vi "main_ctrl.vi"(8 "error in":errorcluster) -> (0 "error out":errorcluster caption="Error")   [LabVIEW 2014]
uses:
  <vilib>/Rock Robotics/WPI/DriverStation/WPI_DriverStationRobotMode2.ctl
  typedefs/test/test data.ctl
  typedefs/test/test controls.ctl
  typedefs/fg_getset.ctl
  typedefs/vision/vision enable.ctl
  typedefs/state machine/subStates.ctl
  typedefs/state machine/singleUseSubstate.ctl
  <vilib>/Rock Robotics/WPI/RobotDrive/WPI_RobotDriveGetSetRefNum.vi
  typedefs/vision/vision data.ctl
  global variables/vision.vi
panel:
  out "vision errors":errorcluster
  in  "Test\nControls":T1 {"Slider" scale=-1.0..1.0}
  out "Test Data":T2
  out "Robot Mode":T3
  out "Vision mSPI":u32
  out "Vision IPS":dbl
  out "Main IPS":dbl
  out "Main mSPI":u32
  # "Test Input/Output"
  # "MAIN CONTROL"
  # "holds robot control code - dual parallel state machine"
  # "mSPI: milliseconds per iteration\nIPS: iterations per second"
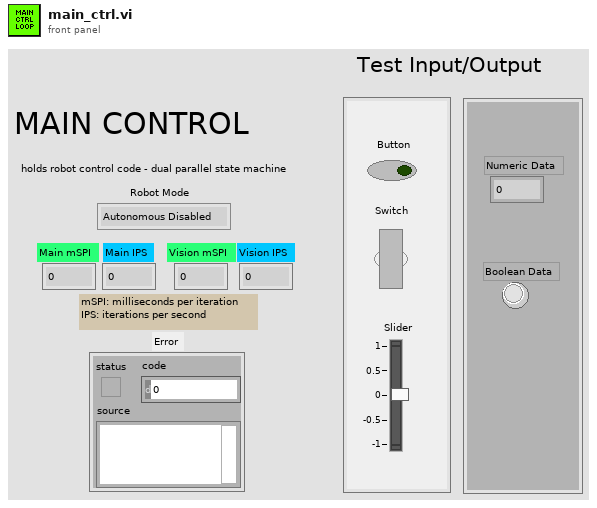
[diagram p1: front panel]
types:
  T1 = typedef "test controls.ctl" = cluster{"Button":bool, "Switch":bool, "Slider":dbl}
  T2 = typedef "test data.ctl" = cluster{"Numeric Data":dbl, "Boolean Data":bool}
  T3 = typedef "WPI_DriverStationRobotMode2.ctl" = enum16{"Autonomous Disabled", "Autonomous Enabled", "Teleop Disabled", "Teleop Enabled", "Disconnected", "Finish", "Test Disabled", "Test Enabled", "Emergency Stopped"}
  T4 = typedef "fg_getset.ctl" = enum16{"Get", "Set"}
  T5 = typedef "vision data.ctl" = cluster{"x":dbl, "y":dbl, "area":dbl, "width":dbl, "height":dbl}
  T6 = typedef "vision enable.ctl" = enum16{"Enable", "Disable", "Stop"}
  T7 = typedef "WPI_CameraDevRef.ctl" = cluster{"Camera Address":string, "CameraStatus":errorcluster}
  T8 = typedef "IMAQ Image.ctl" = refnum<image>
  T9 = typedef "WPI_RobotDriveDevRef.ctl" = cluster{"DevStatus":errorcluster, "Motors[]":T10[], "Square Inputs":bool, "Max Output":dbl}
  T10 = typedef "WPI_MotorControlDeviceRef.ctl" = cluster{"DeviceStatus":errorcluster, "Type":T11, "PWM":cluster{"Controller":T12, "PWM Channel":T13, "DeadBand":T14}, "CAN":cluster{"Device Number":u8, "Control Mode":T15, "Semaphore":T16, "Max Vout":dbl, "TalonSRX Control Mode":T17}, "Invert":bool, "TransformRef":T18, "InvTransformRef":T18}
  T11 = typedef "WPI_MotorControlType.ctl" = enum16{"PWM", "CAN", "CANTalonSRX"}
  T12 = typedef "FPGA_TypedefDigitalModule.ctl" = enum16{"Controller 1"}
  T13 = typedef "FPGA_DIOPWMChannel.ctl" = enum8{"PWM 0", "PWM 1", "PWM 2", "PWM 3", "PWM 4", "PWM 5", "PWM 6", "PWM 7", "PWM 8", "PWM 9", "PWM MXP 0", "PWM MXP 1", "PWM MXP 2", "PWM MXP 3", "PWM MXP 4", "PWM MXP 5", "PWM MXP 6", "PWM MXP 7", "PWM MXP 8", "PWM MXP 9", "Invalid"}
  T14 = typedef "WPI_PWMDeadband.ctl" = cluster{"Name":string, "maxPositivePwm":i32, "minPositivePwm":i32, "centerPwm":i32, "maxNegativePwm":i32, "minNegativePwm":i32, "angularRange":u16}
  T15 = typedef "WPI_CANJaguar_ControlMode.ctl" = enum8{"Percent VBus", "Current", "Speed", "Position", "Voltage"}
  T16 = typedef "Semaphore RefNum" = refnum<k1>
  T17 = typedef "WPI_CANTalonSRX_APIControlMode.ctl" = enum8{"Percent VBus", "Speed", "Position", "Slave", "Unchanged / Invalid"}
  T18 = typedef "WPI_PWMTransform_ConPane.ctl" = refnum<vi>
  T19 = typedef "singleUseSubstate.ctl" = enum16{"null", "wait", "open", "close", "end"}
  T20 = typedef "WPI_DriverStationDerivedRobotMode.ctl" = enum16{"Init", "Execute", "Stop"}
  T21 = typedef "subStates.ctl" = enum16{"null", "wait", "driver control", "auto", "manual override", "hold position", "rotate", "intake", "deposit", "test", "end"}
  T22 = typedef "Loop 2 Datatype.ctl" = cluster{"State":T21, "Waiting Loop":i32, "State to Wait For":i32, "Loop ID":i32, "Exit Value":i32}
  T23 = typedef "Loop 1 Datatype.ctl" = cluster{"State":T21, "Waiting Loop":i32, "State to Wait For":i32, "Loop ID":i32, "Exit Value":i32, "Joystick Y":dbl}
  T24 = typedef "Loop 3 Datatype.ctl" = cluster{"State":T21, "Waiting Loop":i32, "State to Wait For":i32, "Loop ID":i32, "Exit Value":i32, "Speed":dbl}
  T25 = typedef "Loop 0 Datatype.ctl" = cluster{"State":T21, "Waiting Loop":i32, "State to Wait For":i32, "Loop ID":i32, "Exit Value":i32, "X Axis":dbl, "Y Axis":dbl, "Center":dbl, "Mode":enum16{"Arcade Drive", "H-Drive"}}
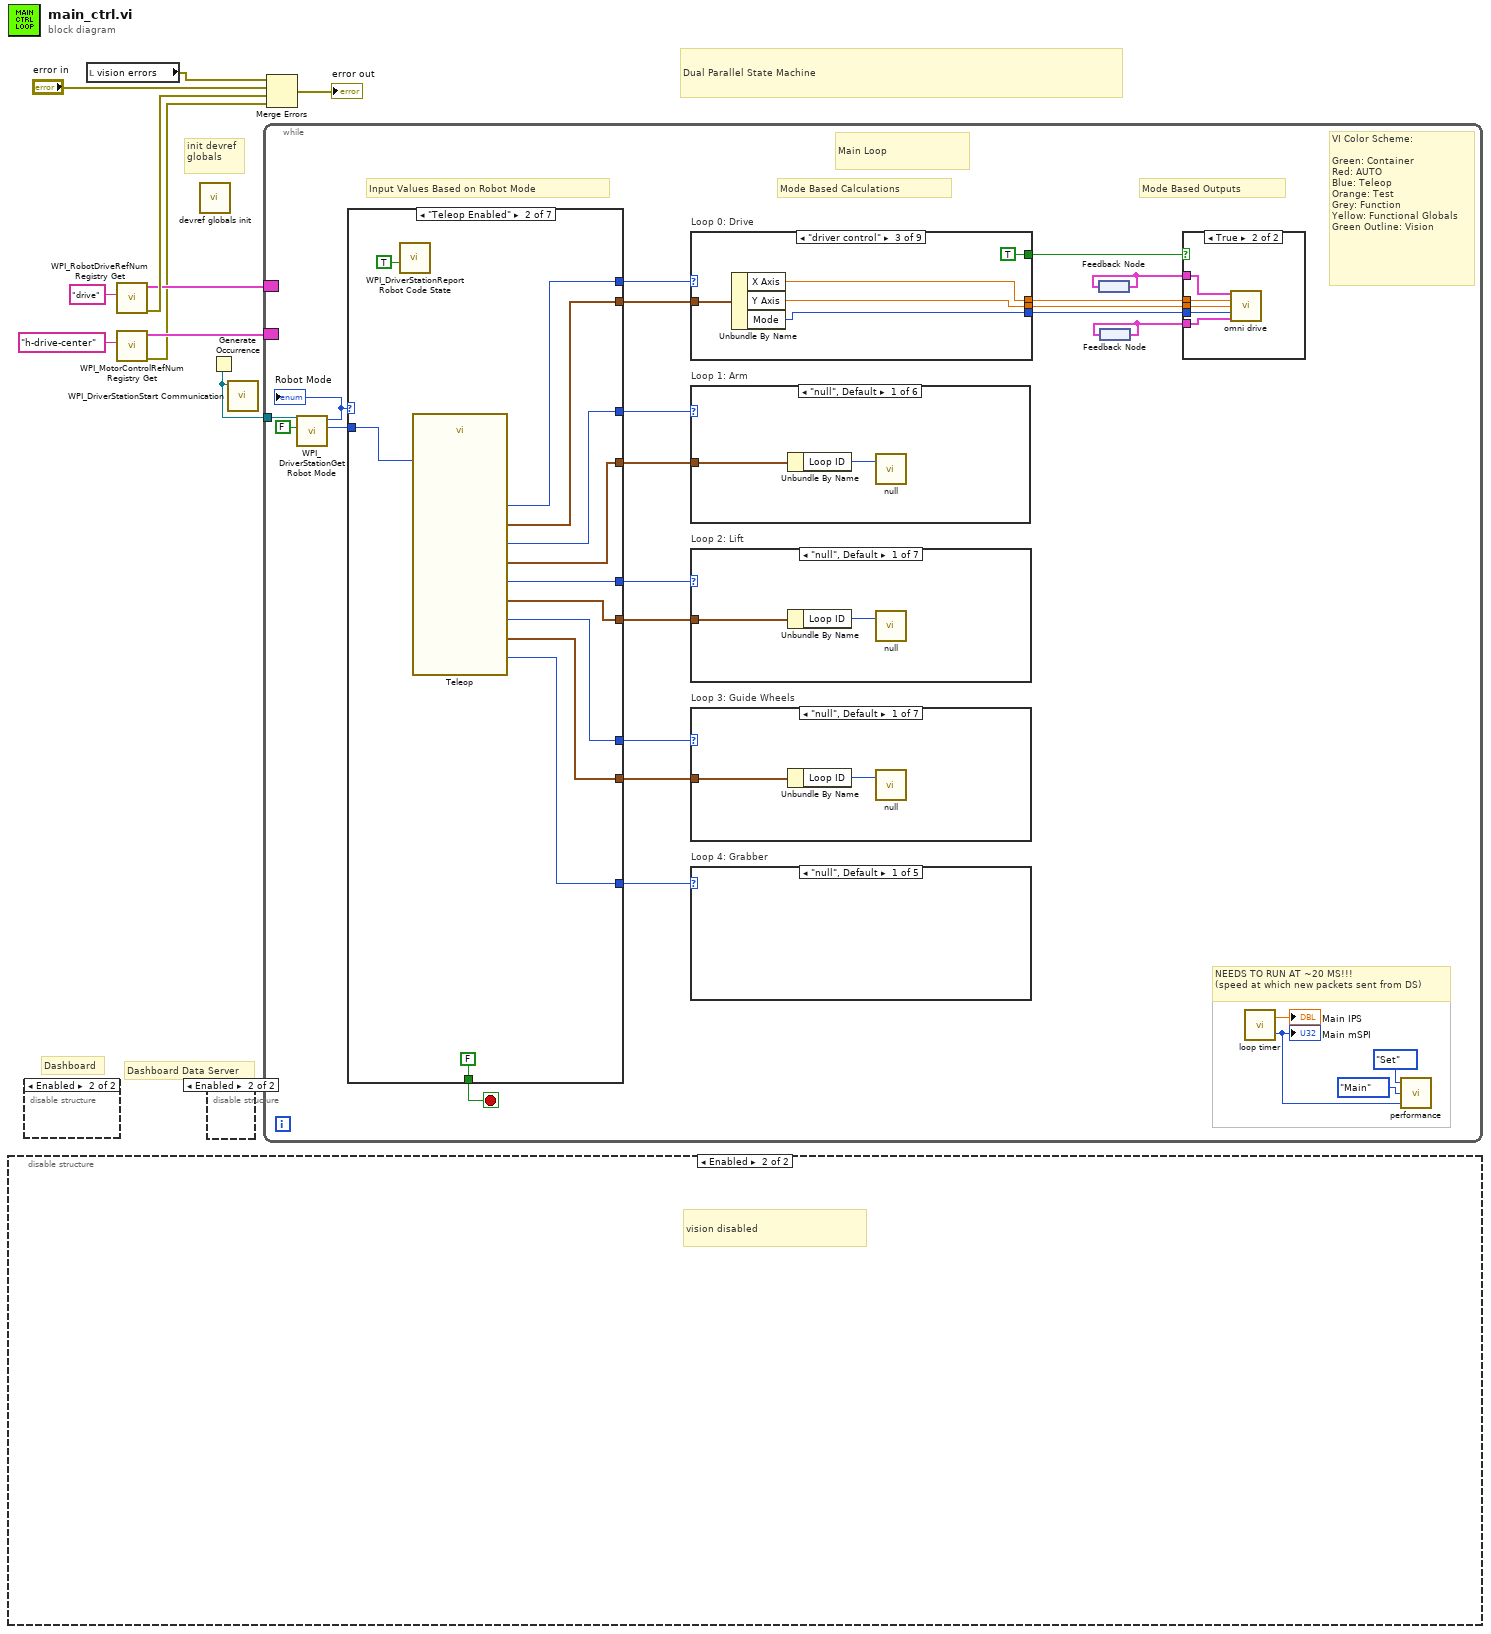
[diagram p0: block diagram]
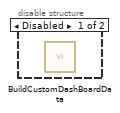
[diagram p2: hidden frame]
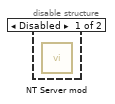
[diagram p3: hidden frame]
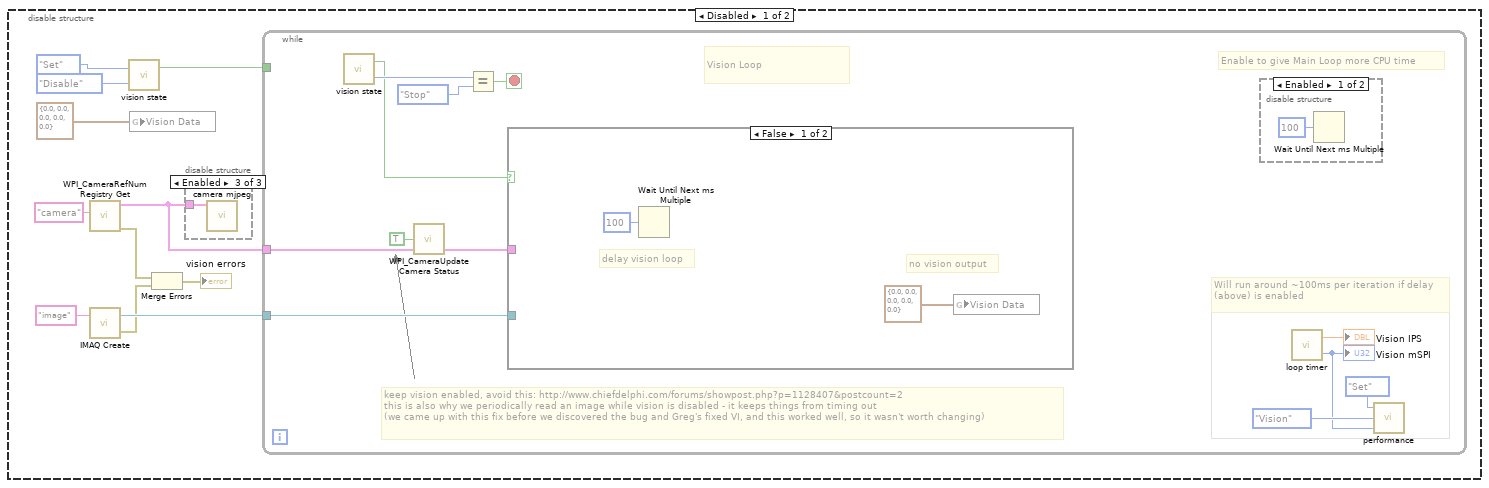
[diagram p4: hidden frame]
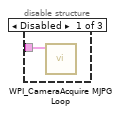
[diagram p5: hidden frame]
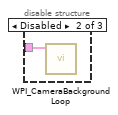
[diagram p6: hidden frame]
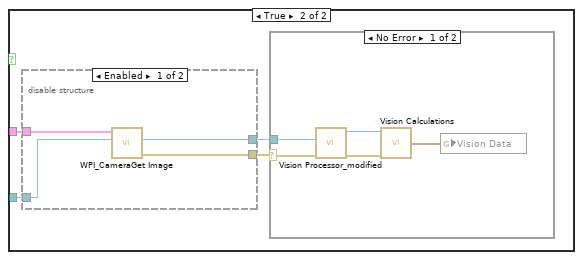
[diagram p8: hidden frame]
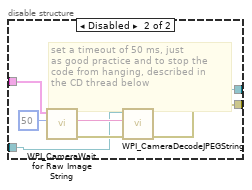
[diagram p10: hidden frame]
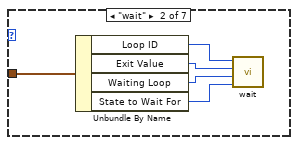
[diagram p15: hidden frame]
diagram:
  # "Dashboard"
  # "init devref\nglobals"
  # "Dual Parallel State Machine"
  # "Dashboard Data Server"
  n1 = disable-structure shown="Enabled" {
    frame Disabled {
      n2 = call <vilib>:"WPI_CameraRefNum Registry Get.vi"("refnum name"="camera") -> ("error out"=w15:errorcluster, "CameraDevRef"=w18:T7)  [unwired: 9 in]
      n3 = call "IMAQ Create"("Image Name"="image") -> ("New Image"=w21:T8, "error out"=w16:errorcluster)  [unwired: 4 in]
      n4 = call "vision state.vi"("State In"=vision_enable."Disable" ("Action"), "Menu"=fg_getset."Set") -> ("Enabled?"=w20:bool)  [unwired: 1 out]
      n5 = global write "vision.vi" "Vision Data"(T5 {"x"=0.0, "y"=0.0, "area"=0.0, "width"=0.0, "height"=0.0} ("Cluster")) -> ()
      n6 = Merge Errors(w15, w16) -> (→"vision errors":errorcluster)
      n7 = disable-structure shown="Enabled" {
        disable-tunnel: w18 -> [w22 w23 w24]
        frame Disabled {
          n8 = call <vilib>:"WPI_CameraAcquire MJPG Loop.vi"("CameraDevRef"=w22) -> ()  [unwired: 11 in]
        }
        frame Disabled {
          n9 = call <vilib>:"WPI_CameraBackground Loop.vi"("CameraDevRef"=w23) -> ()  [unwired: 11 in]
        }
        frame Enabled {
          n10 = call "camera mjpeg.vi"("CameraDevRef"=w24) -> ()  [unwired: 11 in]
        }
      }
      n11 = while {
        tunnel: w21 -> [w35]
        tunnel: w18 -> [w34]
        tunnel: w20 -> [_]
        stop <- w36 stop-if-true
        # "Will run around ~100ms per iteration if delay (above) is enabled"
        # "Enable to give Main Loop more CPU time"
        # "keep vision enabled, avoid this: http://www.chiefdelphi.com/forums/showpost.php?p=1128407&postcount=2\nthis is also why we periodically read an image while vision is disabled - it keeps things from timing out\n(we came up with this fix before we discovered the bug and Greg's fixed VI, and this worked well, so it wasn't worth changing)"
        # "Vision Loop"
        n12 = call "vision state.vi"() -> ("State Out"=w31:T6, "Enabled?"=w27:bool)  [unwired: 2 in]
        n13 = call <vilib>:"WPI_CameraUpdate Camera Status.vi"("CameraDevRef In"=w34, "Enable Vision"=TRUE) -> ("CameraDevRef Out"=w33:T7)  [unwired: 3 in]
        n14 = Equal?(x=w31, y=vision_enable."Stop") -> (x = y?=w36:bool)
        n15 = case shown="False" w27 {
          tunnel: w35 -> [_ w43]
          tunnel: w33 -> [_ w42]
          frame False {
            # "no vision output"
            # "delay vision loop"
            n16 = Wait Until Next ms Multiple(millisecond multiple=u32 100) -> ()  [unwired: 1 out]
            n17 = global write "vision.vi" "Vision Data"(T5 {"x"=0.0, "y"=0.0, "area"=0.0, "width"=0.0, "height"=0.0} ("Cluster")) -> ()
          }
          frame True {
            n18 = disable-structure shown="Enabled" {
              disable-tunnel: w43 -> [w51 w55]
              disable-tunnel: w42 -> [w52 w57]
              disable-tunnel: [w50 w54] -> w41
              disable-tunnel: [w49 w53] -> w40
              frame Enabled {
                n19 = call <vilib>:"WPI_CameraGet Image.vi"("Image"=w51, "CameraDevRef"=w52) -> ("error out"=w49:errorcluster, "Image Out"=w50:T8)  [unwired: 7 in, 1 out]
              }
              frame Disabled {
                # "set a timeout of 50 ms, just\nas good practice and to stop the \ncode from hanging, described in \nthe CD thread below"
                n20 = call <vilib>:"WPI_CameraWait for Raw Image String.vi"("Timeout in ms (-1)"=50, "CameraDevRef"=w57) -> ("error out"=w59:errorcluster, "String"=w58:string)  [unwired: 3 in, 5 out]
                n21 = call <vilib>:"WPI_CameraDecodeJPEGString.vi"("error in"=w59, "Compressed Image"=w58, "Image In"=w55) -> ("error out"=w53:errorcluster, "Image Out"=w54:T8)  [unwired: 3 out]
              }
            }
            n22 = case shown="No Error" w40 {
              selector: w40 -> [w48 _]
              tunnel: w41 -> [w47 _]
              frame No Error {
                n23 = call "Vision Processor_modified.vi"("error in"=w48, "Image In"=w47) -> ("error out"=w45:errorcluster, "Image Out"=w46:T8)  [unwired: 5 in]
                n24 = call "Vision Calculations.vi"("Image In"=w46, "error in"=w45) -> ("Vision Data"=w44:T5)  [unwired: 3 in]
                n25 = global write "vision.vi" "Vision Data"(w44) -> ()
              }
              frame Error {
              }
            }
          }
        }
        n26 = disable-structure shown="Enabled" {
          frame Enabled {
            n27 = Wait Until Next ms Multiple(millisecond multiple=u32 100) -> ()  [unwired: 1 out]
          }
          frame Disabled {
          }
        }
        n28 = call "loop timer.vi"() -> ("IPS"=→"Vision IPS":dbl, "mSPI"=w25:u32)  [unwired: 1 in]
        "Vision mSPI" <- w25
        n29 = call "performance.vi"("mSPI"=w25, "Loop"=enum16{"Main", "Vision", "Dash"}."Vision", "Menu"=fg_getset."Set") -> ()  [unwired: 1 out]
      }
    }
    frame Enabled {
      # "vision disabled"
    }
  }
  n30 = disable-structure shown="Enabled" {
    frame Disabled {
      n31 = call "BuildCustomDashBoardData.vi"() -> ()  [unwired: 12 in]
    }
    frame Enabled {
    }
  }
  n32 = local read "vision errors"() -> (w6:errorcluster)
  n33 = call <vilib>:"WPI_RobotDriveRefNum Registry Get.vi"("refnum name"="drive") -> ("error out"=w5:errorcluster, "RobotDriveDevRef"=w2:T9)  [unwired: 9 in]
  n34 = call <vilib>:"WPI_MotorControlRefNum Registry Get.vi"("refnum name"="h-drive-center") -> ("error out"=w1:errorcluster, "MotorControlDevRef"=w3:T10)  [unwired: 9 in]
  n35 = call "devref globals init.vi"() -> ()  [unwired: 12 in]
  n36 = disable-structure shown="Enabled" {
    frame Disabled {
      n37 = call "NT Server mod.vi"() -> ()  [unwired: 12 in]
    }
    frame Enabled {
    }
  }
  n38 = Generate Occurrence() -> (w8:refnum<k4>)
  n39 = call <vilib>:"WPI_DriverStationStart Communication.vi"("occurrence"=w8) -> ()  [unwired: 11 in]
  n40 = while {
    tunnel: w8 -> [w73]
    border: w2 -> [_]
    border: w3 -> [_]
    stop <- w81 stop-if-true
    # "Mode Based Outputs"
    # "VI Color Scheme:\n\nGreen: Container\nRed: AUTO\nBlue: Teleop\nOrange: Test \nGrey: Function\nYellow: Functional Globals\nGreen Outline: Vision"
    # "Input Values Based on Robot Mode"
    # "Mode Based Calculations"
    # "NEEDS TO RUN AT ~20 MS!!!\n(speed at which new packets sent from DS)"
    # "Main Loop"
    n41 = call <vilib>:"WPI_DriverStationGet Robot Mode.vi"("Finish"=FALSE, "DS Occurrence"=w73) -> ("Call Context"=w72:T20, "Robot Mode"=w71:T3)  [unwired: 8 out]
    "Robot Mode" <- w71
    n42 = case shown="\"Teleop Enabled\"" w71 {
      tunnel: [w163 w178 w188 w194 w200 w202 w206] -> w75
      tunnel: w72 -> [w157 w175 w180 _ _ _ _]
      tunnel: [w161 w177 w190 w194 w200 w202 w206] -> w82
      tunnel: [FALSE FALSE FALSE FALSE FALSE FALSE TRUE] -> w81
      tunnel: [w165 w174 w186 w194 w200 w202 w206] -> w70
      tunnel: [w164 w173 w187 _ _ _ _] -> w80
      tunnel: [w162 w172 w189 _ _ _ _] -> w79
      tunnel: [w160 w171 w185 _ _ _ _] -> w78
      tunnel: [w158 w170 w183 _ _ _ _] -> w66
      tunnel: [w159 w169 w184 w194 w200 w202 w206] -> w67
      tunnel: [w155 w167 w179 singleUseSubstate."null" ("SubState 5") singleUseSubstate."null" ("SubState 5") singleUseSubstate."null" ("SubState 5") singleUseSubstate."null" ("SubState 5")] -> w65
      frame "Autonomous Enabled" {
        n43 = call <vilib>:"WPI_DriverStationReport Robot Code State.vi"("Autonomous"=TRUE) -> ()  [unwired: 10 in, 1 out]
        n44 = call "Autonomous.vi"("Call Context"=w157) -> ("SubState 2"=w161:T21, "Loop 2 Data"=w160:T22, "SubState 1"=w163:T21, "Loop 1 Data"=w162:T23, "Loop 3 Data"=w158:T24, "SubState 0"=w165:T21, "SubState 3"=w159:T21, "Loop 0 Data"=w164:T25, "SubState 4"=w155:T19)  [unwired: 2 in]
      }
      frame "Teleop Enabled" {
        n45 = call <vilib>:"WPI_DriverStationReport Robot Code State.vi"("TeleOp"=TRUE) -> ()  [unwired: 10 in, 1 out]
        n46 = call "Teleop.vi"("Call Context"=w175) -> ("SubState 3"=w169:T21, "Loop 3 Data"=w170:T24, "SubState 4"=w167:T19, "SubState 0"=w174:T21, "Loop 1 Data"=w172:T23, "Loop 0 Data"=w173:T25, "SubState 1"=w178:T21, "Loop 2 Data"=w171:T22, "SubState 2"=w177:T21)  [unwired: 10 in]
      }
      frame "Test Enabled" {
        n47 = call "test io.vi"("Call Context"=w180) -> ("Test Data"=→"Test Data":T2)
        n48 = call <vilib>:"WPI_DriverStationReport Robot Code State.vi"("Test"=TRUE) -> ()  [unwired: 10 in, 1 out]
        n49 = call "Test.vi"("Call Context"=w180, "Test Controls"="Test\nControls") -> ("SubState 0"=w186:T21, "Loop 0 Data"=w187:T25, "SubState 1"=w188:T21, "Loop 1 Data"=w189:T23, "SubState 2"=w190:T21, "SubState 4"=w179:T19, "Loop 3 Data"=w183:T24, "SubState 3"=w184:T21, "Loop 2 Data"=w185:T22)  [unwired: 5 in]
      }
      frame "Autonomous Disabled", "Teleop Disabled", "Test Disabled" {
        w194 = subStates."null" ("SubState 0")
        (unwired) fg_getset."Set" ("Menu")
        # "set all loops to null"
        # "make sure to disable vision\nwe don't need it here"
        # "Robot Disabled"
        n50 = call <vilib>:"WPI_DriverStationReport Robot Code State.vi"("Disabled"=TRUE) -> ()  [unwired: 10 in, 1 out]
        n51 = call "vision state.vi"("State In"=vision_enable."Disable" ("Action")) -> ()  [unwired: 1 in, 2 out]
      }
      frame "Disconnected" {
        w200 = subStates."null" ("Loop State")
        # "Potential Debugging Time\naccording to the example code\n\nmaybe run the test i/o VI?"
      }
      frame "Emergency Stopped" {
        w202 = subStates."null" ("Loop State")
        # "Well this can't be good...\n\nwe can use this case for something or\nappend it to the series of disabled cases"
      }
      frame "Finish" {
        w206 = subStates."end" ("Loop State")
        # "stop vision loop"
        # "Stop All Loops"
        # "stop the while loop"
        n52 = call "vision state.vi"("State In"=vision_enable."Stop" ("Action"), "Menu"=fg_getset."Set") -> ()  [unwired: 2 out]
      }
    }
    n53 = case "Loop 0: Drive" shown="\"driver control\"" w70 {
      tunnel: w80 -> [w106 w109 w118 w124 w132 w134 w141 _ _]
      tunnel: [w105 w108 w117 w121 w129 w136 w143 w144 w147] -> w69
      tunnel: [w105 w108 w116 w120 w128 w135 w142 w144 w147] -> w68
      tunnel: [FALSE FALSE TRUE FALSE FALSE FALSE FALSE TRUE FALSE] -> w77
      tunnel: [_ _ w114 _ _ _ _ _ _] -> w60
      frame "null", Default {
        w105 = 0.0 ("X Axis")
        n54 = Unbundle By Name(w106) -> ("Loop ID"=w103:i32)
        n55 = call "null.vi"("This Loop ID"=w103) -> ()  [unwired: 2 in]
      }
      frame "wait" {
        w108 = 0.0 ("X Axis")
        n56 = Unbundle By Name(w109) -> ("Loop ID"=w113:i32, "Exit Value"=w112:i32, "Waiting Loop"=w111:i32, "State to Wait For"=w110:i32)
        n57 = call "wait.vi"("State to wait for"=w110, "Waiting Loop ID"=w111, "Time (ms)"=w112, "Current Loop ID"=w113) -> ()  [unwired: 1 out]
      }
      frame "driver control" {
        n58 = Unbundle By Name(w118) -> ("X Axis"=w117:dbl, "Y Axis"=w116:dbl, "Mode"=w114:enum16{"Arcade Drive", "H-Drive"})
      }
      frame "manual override" {
        n59 = Unbundle By Name(w124) -> ("X Axis"=w123:dbl, "Y Axis"=w122:dbl)
        n60 = expression code="x/2"(w123) -> (w121:dbl)
        n61 = expression code="x/2"(w122) -> (w120:dbl)
      }
      frame "hold position" {
        n62 = Unbundle By Name(w132) -> ("X Axis"=w131:dbl, "Y Axis"=w130:dbl)
        n63 = call "closed hold.vi"("Acrade Drive?"=TRUE, "Y axis value (Left)"=w130, "X axis value (Right)"=w131, "Threshold (.4)"=0.4) -> ("right"=w128:dbl, "left"=w129:dbl)
      }
      frame "auto" {
        n64 = Unbundle By Name(w134) -> ("X Axis"=w133:dbl)
        n65 = call "autoDrive.vi"("Distance"=w133) -> ("right speed"=w135:dbl, "left speed"=w136:dbl)  [unwired: 2 in, 1 out]
      }
      frame "rotate" {
        n66 = Unbundle By Name(w141) -> ("X Axis"=w140:dbl, "Y Axis"=w139:dbl)
        n67 = call "rotate.vi"("Rate"=w139, "Angle"=w140) -> ("right speed"=w142:dbl, "left speed"=w143:dbl)  [unwired: 1 in, 1 out]
      }
      frame "test" {
        w144 = 0.0
      }
      frame "end" {
        w147 = 0.0 ("X Axis")
      }
    }
    n68 = case "Loop 1: Arm" shown="\"null\", Default" w75 {
      tunnel: w79 -> [w149 w150 _ _ _ _]
      frame "null", Default {
        n69 = Unbundle By Name(w149) -> ("Loop ID"=w148:i32)
        n70 = call "null.vi"("This Loop ID"=w148) -> ()  [unwired: 2 in]
      }
      frame "wait" {
        n71 = Unbundle By Name(w150) -> ("Loop ID"=w154:i32, "Exit Value"=w153:i32, "Waiting Loop"=w152:i32, "State to Wait For"=w151:i32)
        n72 = call "wait.vi"("State to wait for"=w151, "Waiting Loop ID"=w152, "Time (ms)"=w153, "Current Loop ID"=w154) -> ()  [unwired: 1 out]
      }
      frame "auto" {
      }
      frame "manual override" {
      }
      frame "test" {
      }
      frame "end" {
      }
    }
    n73 = case "Loop 2: Lift" shown="\"null\", Default" w82 {
      tunnel: w78 -> [w92 w93 _ _ _ _ _]
      frame "null", Default {
        n74 = Unbundle By Name(w92) -> ("Loop ID"=w91:i32)
        n75 = call "null.vi"("This Loop ID"=w91) -> ()  [unwired: 2 in]
      }
      frame "wait" {
        n76 = Unbundle By Name(w93) -> ("Loop ID"=w97:i32, "Exit Value"=w96:i32, "Waiting Loop"=w95:i32, "State to Wait For"=w94:i32)
        n77 = call "wait.vi"("State to wait for"=w94, "Waiting Loop ID"=w95, "Time (ms)"=w96, "Current Loop ID"=w97) -> ()  [unwired: 1 out]
      }
      frame "driver control" {
      }
      frame "manual override" {
      }
      frame "auto" {
      }
      frame "test" {
      }
      frame "end" {
      }
    }
    n78 = case "Loop 3: Guide Wheels" shown="\"null\", Default" w67 {
      tunnel: w66 -> [w85 w86 _ _ _ _ _]
      frame "null", Default {
        n79 = Unbundle By Name(w85) -> ("Loop ID"=w84:i32)
        n80 = call "null.vi"("This Loop ID"=w84) -> ()  [unwired: 2 in]
      }
      frame "wait" {
        n81 = Unbundle By Name(w86) -> ("Loop ID"=w90:i32, "Exit Value"=w89:i32, "Waiting Loop"=w88:i32, "State to Wait For"=w87:i32)
        n82 = call "wait.vi"("State to wait for"=w87, "Waiting Loop ID"=w88, "Time (ms)"=w89, "Current Loop ID"=w90) -> ()  [unwired: 1 out]
      }
      frame "driver control" {
      }
      frame "manual override" {
      }
      frame "auto" {
      }
      frame "test" {
      }
      frame "end" {
      }
    }
    n83 = case "Loop 4: Grabber" shown="\"null\", Default" w65 {
      frame "null", Default {
      }
      frame "wait" {
      }
      frame "open" {
      }
      frame "close" {
      }
      frame "end" {
      }
    }
    n84 = feedback #1() -> (w76:T9)
    n85 = feedback-in #1(w76) -> ()
    n86 = feedback #2() -> (w61:T10)
    n87 = feedback-in #2(w61) -> ()
    n88 = case shown="True" w77 {
      tunnel: w69 -> [_ w100]
      tunnel: w68 -> [_ w102]
      tunnel: w76 -> [_ w99]
      tunnel: w61 -> [_ w101]
      tunnel: w60 -> [_ w98]
      frame False {
      }
      frame True {
        n89 = call "omni drive.vi"("Drive RefNum"=w99, "X Axis"=w100, "Y Axis"=w102, "Drive Mode"=w98, "Center Motor"=w101) -> ()  [unwired: 11 in]
      }
    }
    n90 = call "loop timer.vi"() -> ("IPS"=→"Main IPS":dbl, "mSPI"=w63:u32)  [unwired: 1 in]
    "Main mSPI" <- w63
    n91 = call "performance.vi"("mSPI"=w63, "Loop"=enum16{"Main", "Vision", "Dash"}."Main", "Menu"=fg_getset."Set") -> ()  [unwired: 1 out]
  }
  n92 = Merge Errors(w6, "error in", w5, w1) -> (→"error out":errorcluster)
